vi "ESC Set RPM With Calib oneshot.vi"(3 "Error In":errorcluster, 4 "Calib File":path, 5 "Desired RPM":dbl min=0.0 max=15100.0) -> (0 "Error out":errorcluster, 2 "PWM%":dbl format="%.2f")   [LabVIEW 2021]
uses:
  Anemometry/Anemometry Sub Vis/Controls/Inst_type.ctl
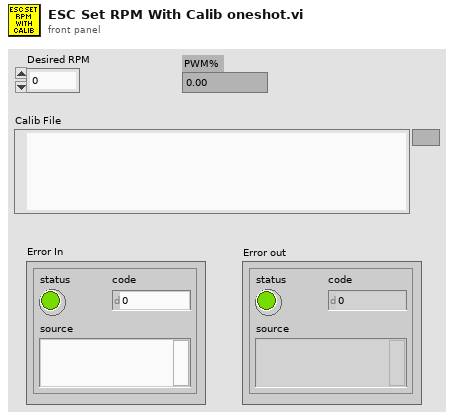
[diagram p1: front panel]
types:
  T1 = typedef "Inst_type.ctl" = enum16{"Raw voltage", "Raw with zero offsetting", "Propeller anemometer", "Pressure Transducer", "Pitot-static tube", "Hot wire", "Cross wire 1", "Cross wire 2", "Generic Linear", "Generic Polynomial", "Generic BackPoly", "Fast FID", "Thermocouple", "Cold wire", "Pulsed Wire", "LDA Vel", "LDA Tran time", "LDA Arr time", "Microphone"}
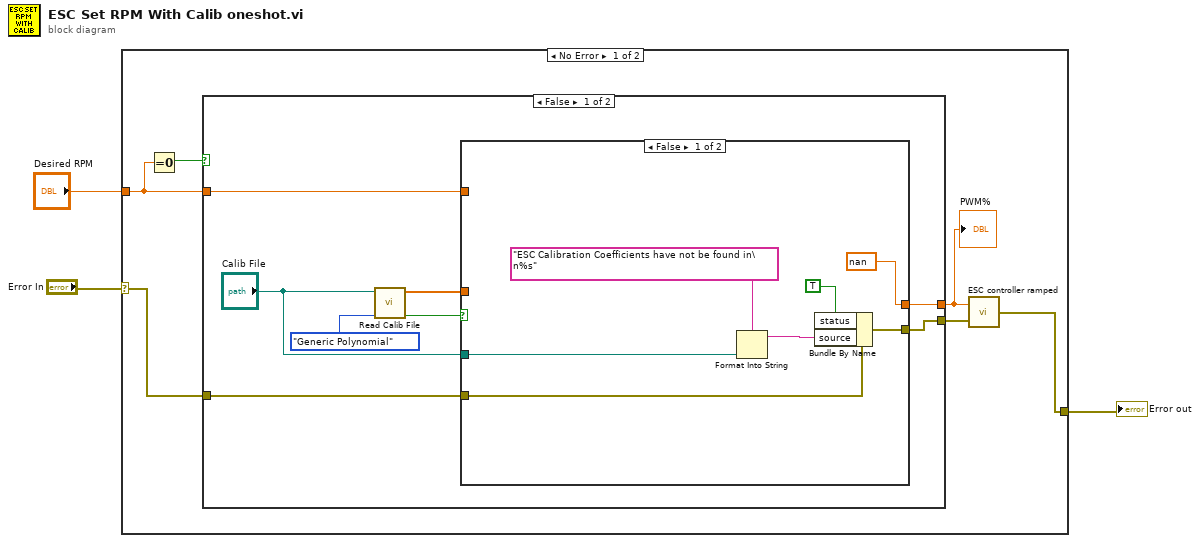
[diagram p0: block diagram]
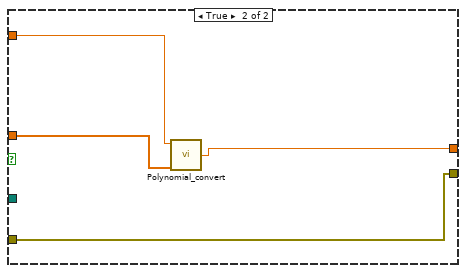
[diagram p2: hidden frame]
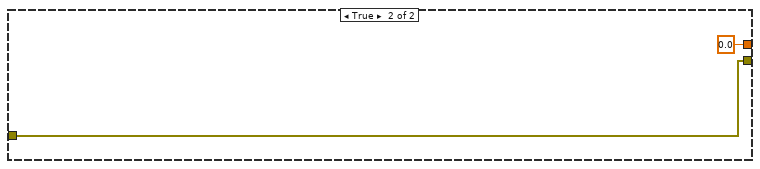
[diagram p3: hidden frame]
diagram:
  n1 = case shown="No Error" "Error In" {
    selector: "Error In" -> [w9 w31]
    tunnel: [w8 w31] -> w3
    tunnel: "Desired RPM" -> [w6 _]
    frame No Error {
      n2 = Equal To 0?(x=w6) -> (x = 0?=w5:bool)
      n3 = case shown="False" w5 {
        tunnel: w9 -> [w15 w29]
        tunnel: [w12 0.0 ("Eng Values")] -> w4
        tunnel: [w11 w29] -> w7
        tunnel: w6 -> [w10 _]
        frame False {
          n4 = call "Read Calib File.vi"("Inst type"=Inst_type."Generic Polynomial", "Calib File"="Calib File") -> ("Coefficients Found?"=w17:bool, "Calib Constants"=w16:dbl[])  [unwired: 8 in]
          n5 = case shown="False" w17 {
            tunnel: w10 -> [_ w28]
            tunnel: w16 -> [_ w27]
            tunnel: [w22 w25] -> w11
            tunnel: w15 -> [w24 w25]
            tunnel: "Calib File" -> [w21 _]
            tunnel: [nan w26] -> w12
            frame False {
              n6 = Format Into String(format string="ESC Calibration Coefficients have not be found in\n%s", w21) -> (resulting string=w20:string)  [unwired: 2 in, 1 out]
              n7 = Bundle By Name(cluster=w24, "status"=TRUE, "source"=w20) -> (w22:errorcluster)
            }
            frame True {
              n8 = call "Polynomial_convert.vi"("Calib constants"=w27, "Voltage"=w28) -> ("Eng Values"=w26:dbl)  [unwired: 4 out]
            }
          }
        }
        frame True {
        }
      }
      "PWM%" <- w4
      n9 = call "ESC controller ramped.vi"("Error In"=w7, "Output %"=w4) -> ("Error out"=w8:errorcluster)  [unwired: 1 in]
    }
    frame Error {
    }
  }
  "Error out" <- w3
